vi "Servicio to contabilidad.vi"(8 "error in (no error)":errorcluster, 10 "Servicio seleccionado":string, 11 "UI in":refnum<class "UI.lvclass">) -> (0 "error out":errorcluster, 3 "UI out":refnum<class "UI.lvclass">)   [LabVIEW 2020, in "UI.lvlib" / "UI.lvclass"]
uses:
  UI.lvclass
  UI.lvclass/UI.ctl
  Contabilidad Messages/Get servicio from ui Msg/Get servicio from ui Msg.lvclass/Get servicio from ui Msg.ctl
  <vilib>/ActorFramework/Message Enqueuer/Message Enqueuer.lvclass/Message Enqueuer.ctl
  <vilib>/ActorFramework/Message Enqueuer/Enqueue.vi
  Contabilidad Messages/Get servicio from ui Msg/Get servicio from ui Msg.lvclass
  C:/Program Files (x86)/National Instruments/LabVIEW 2020/vi.lib/ActorFramework/Message/Message.lvclass
  <vilib>/ActorFramework/Message Priority Queue/Priority Enqueue.vi
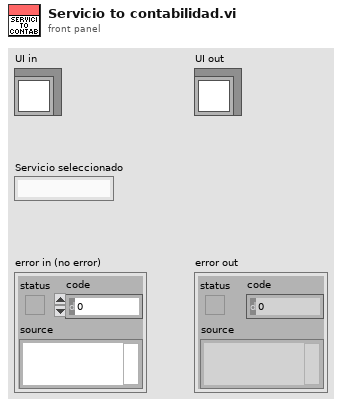
[diagram p1: front panel]
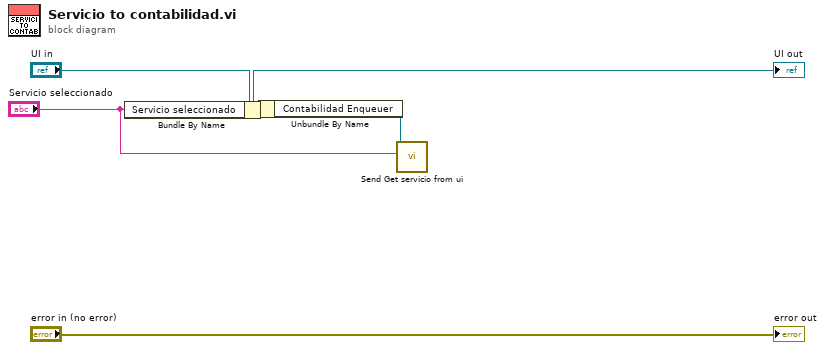
[diagram p0: block diagram]
diagram:
  n1 = Bundle By Name(cluster="UI in", "Servicio seleccionado"="Servicio seleccionado") -> (w2:refnum<class "UI.lvclass">)
  "UI out" <- w2
  n2 = Unbundle By Name(w2) -> ("Contabilidad Enqueuer"=w1:refnum<class "Message Enqueuer.lvclass">)
  n3 = call "Send Get servicio from ui.vi"("Servicio seleccionado"="Servicio seleccionado", "Message Enqueuer"=w1) -> ()  [unwired: 8 in, 2 out]
  "error out" <- "error in (no error)"
